vi "readSerial.vi"(9 "baud rate (9600)":u32=9600, 10 "VISA resource name":refnum<visa-resource-name>) -> (2 "read buffer":string)   [LabVIEW 2023]
uses:
  <vilib>/Instr/_visa.llb/VISA Configure Serial Port (Instr).vi
panel:
  in  "byte count":u32
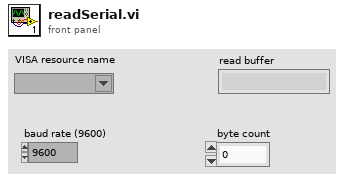
[diagram p1: front panel]
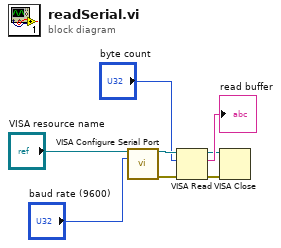
[diagram p0: block diagram]
diagram:
  n1 = call-poly "VISA Configure Serial Port"("VISA resource name"="VISA resource name", "baud rate (9600)"="baud rate (9600)") -> ("VISA resource name out"=w7:refnum<visa-resource-name>, "error out"=w8:errorcluster)  [unwired: 12 in]
  n2 = VISA Read(VISA resource name=w7, byte count="byte count", error in (no error)=w8) -> (VISA resource name out=w1:refnum<visa-resource-name>, read buffer=→"read buffer":string, error out=w2:errorcluster)  [unwired: 1 out]
  n3 = VISA Close(VISA resource name=w1, error in (no error)=w2) -> ()  [unwired: 1 out]
